vi "FFT_amplitude_phsae.vi"() -> ()   [LabVIEW 2017]
uses:
  <vilib>/measure/maspectr.llb/FFT Spectrum (Real-Im) for 1 Chan.vi
  <vilib>/measure/NI_MABase.lvlib
  <vilib>/measure/NI_MAPro.lvlib
panel:
  out "Phase Spectrum":dbl[](graph)
  out "웨이브폼 그래프 3":cluster{"f0":dbl, "df":dbl, dbl[]}(graph)
  out "웨이브폼 그래프 2":cluster{"f0":dbl, "df":dbl, dbl[]}(graph)
  out "웨이브폼 그래프":waveform(dbl)(graph)
  in  "sampling info":cluster{"Fs":dbl, "#s":dbl}={"Fs"=1000.0, "#s"=1000.0} caption="샘플링 정보" {"Fs" format="%.2p"}
  in  "phase":dbl caption="위상" format="%.2p"
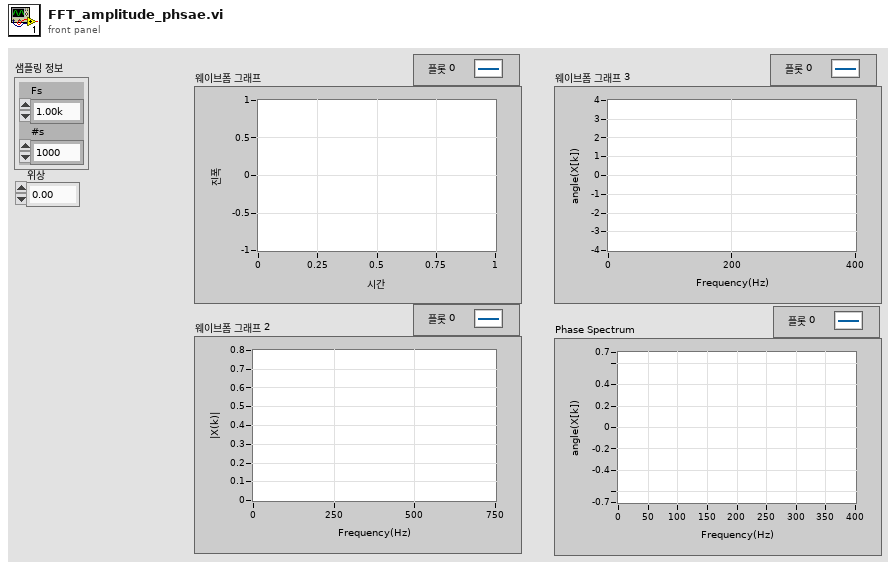
[diagram p1: front panel]
types:
  T1 = cluster{"f0":dbl, "df":dbl, "imaginary part":dbl[]}
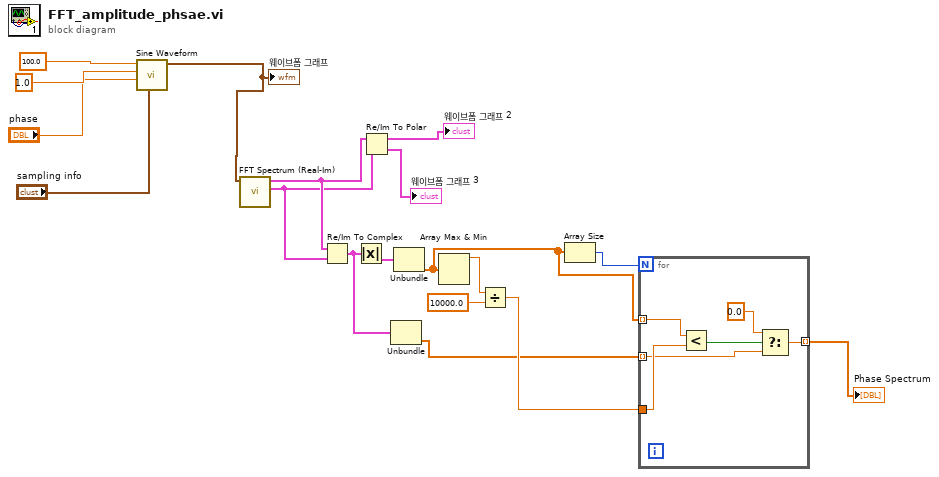
[diagram p0: block diagram]
diagram:
  n1 = call <vilib>:"Sine Waveform.vi"("sampling info"="sampling info", "phase"="phase", "amplitude"=1.0, "frequency"=100.0) -> ("signal out"=w14:waveform(dbl))  [unwired: 6 in, 1 out]
  "웨이브폼 그래프" <- w14
  n2 = call-poly <vilib>:"FFT Spectrum (Real-Im).vi"("time signal"=w14) -> ("imaginary part"=w10:T1, "real part"=w11:cluster{"f0":dbl, "df":dbl, "real part":dbl[]})  [unwired: 6 in, 3 out]
  n3 = Re/Im To Complex(1:w10, 2:w11) -> (0:w2:cluster{"f0":cdb, "df":cdb, cdb[]})
  n4 = Absolute Value(x=w2) -> (abs(x)=w6:cluster{"f0":dbl, "df":dbl, dbl[]})
  n5 = Re/Im To Polar(2:w10, 3:w11) -> (0:→"웨이브폼 그래프 3":cluster{"f0":dbl, "df":dbl, dbl[]}, 1:→"웨이브폼 그래프 2":cluster{"f0":dbl, "df":dbl, dbl[]})
  n6 = Unbundle(w2) -> (w1:cdb[])  [unwired: 2 out]
  n7 = Unbundle(w6) -> (w3:dbl[])  [unwired: 2 out]
  n8 = Array Max & Min(array=w3) -> (max value=w9:dbl)  [unwired: 3 out]
  n9 = Divide(x=w9, y=10000.0) -> (x/y=w4:dbl)
  n10 = Array Size(array=w3) -> (size(s)=w5:i32)
  n11 = for {
    N: w5 -> [_]
    tunnel: w4 -> [w24]
    tunnel: w3 -> [w21] mode=indexing
    tunnel: [w20] -> w7 mode=indexing
    tunnel: w1 -> [w19] mode=indexing
    n12 = Less?(x=w21, y=w24) -> (x < y?=w23:bool)
    n13 = Select(t=0.0, s=w23, f=w19) -> (s? t:f=w20:cdb)
  }
  "Phase Spectrum" <- w7
